vi "限幅器（I64）.vi"(3 "下限":i64, 4 "X_in":i64, 5 "上限":i64) -> (1 "X_Out":i64)   [LabVIEW 2012]
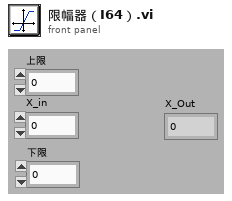
[diagram p1: front panel]
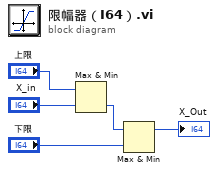
[diagram p0: block diagram]
diagram:
  n1 = Max & Min(x="上限", y="X_in") -> (min(x,y)=w3:i64)  [unwired: 1 out]
  n2 = Max & Min(x=w3, y="下限") -> (max(x,y)=→"X_Out":i64)  [unwired: 1 out]
